vi "Check if no Measurement Selected.vi"(8 "error in (no error)":errorcluster, 11 "multicolumnListbox in":refnum<vi>) -> (0 "error out":errorcluster, 1 "warning?":string, 2 "create client disabled?":T1(ring), 3 "multicolumnListbox out":refnum<vi>)   [LabVIEW 2021, in "MeasurementClient Editor.lvlib"]
uses:
  MeasurementClient Editor.lvlib
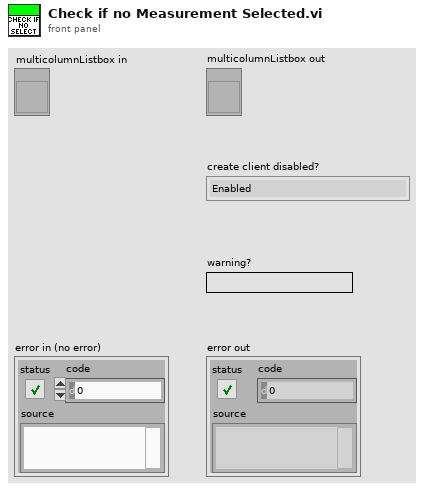
[diagram p1: front panel]
types:
  T1 = enum8{"Enabled", "Disabled", "Disabled and Grayed Out"}
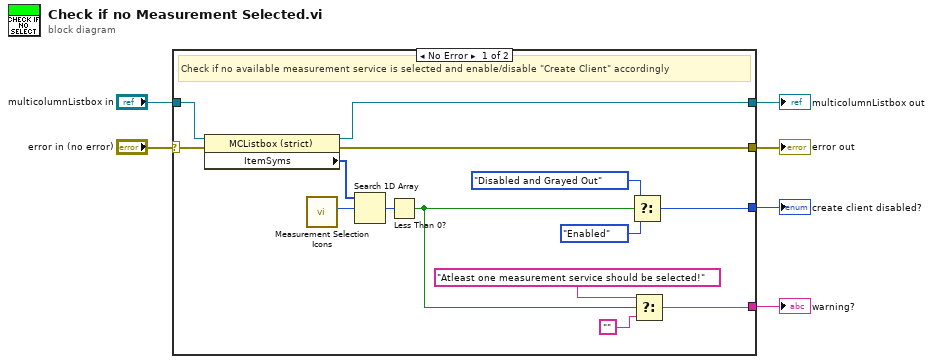
[diagram p0: block diagram]
diagram:
  n1 = case shown="No Error" "error in (no error)" {
    selector: "error in (no error)" -> [w14 w21]
    tunnel: "multicolumnListbox in" -> [w16 w22]
    tunnel: [w15 w21] -> w5
    tunnel: [w13 _] -> w3
    tunnel: [w12 w22] -> w2
    tunnel: [w7 _] -> w1
    frame No Error {
      # "Check if no available measurement service is selected and enable/disable \"Create Client\" accordingly"
      n2 = property class="MCListbox (strict)"(reference=w16, error in=w14) -> (reference out=w12:refnum<vi>, error out=w15:errorcluster, "ItemSyms"=w17:i32[])
      n3 = call "Measurement Selection Icons.vi"() -> ("Checked"=w11:i32)  [unwired: 10 in, 1 out]
      n4 = Search 1D Array(1D array=w17, element=w11) -> (index of element=w18:i32)  [unwired: 1 in]
      n5 = Less Than 0?(x=w18) -> (x < 0?=w8:bool)
      n6 = Select(t=T1."Disabled and Grayed Out", s=w8, f=T1."Enabled" ("Disabled")) -> (s? t:f=w13:T1)
      n7 = Select(t="Atleast one measurement service should be selected!", s=w8, f="") -> (s? t:f=w7:string)
    }
    frame Error {
      # "Pass"
    }
  }
  "error out" <- w5
  "create client disabled?" <- w3
  "multicolumnListbox out" <- w2
  "warning?" <- w1
